vi "Search 1D Array -placeContent.vi"   [LabVIEW 2017]
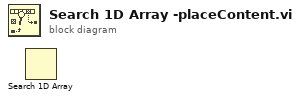
[diagram p0: block diagram]
diagram:
  n1 = Search 1D Array() -> ()  [unwired: 3 in, 1 out]
